vi "Create_LV_INI_Token.vi"   [LabVIEW 2021]
uses:
  <vilib>/Utility/config.llb/Write Key (String).vi
  <vilib>/Wiresmith Technology/G CLI/CLI Class/CLI.lvclass
  <vilib>/Utility/config.llb/NI_LVConfig.lvlib
types:
  T1 = enum32{"Invalid", "Standard", "Closed", "Hidden", "Minimized", "Maximized"}
  T2 = typedef "NI_LVConfig.lvlib/Config Data RefNum.ctl" = refnum<k1>
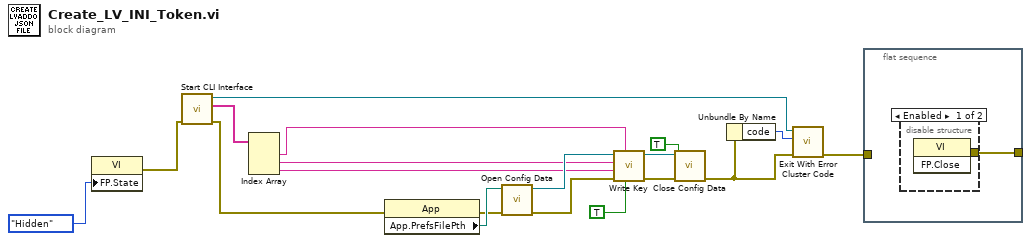
[diagram p0: block diagram]
diagram:
  n1 = property class="VI"("FP.State"=T1."Hidden" ("Front Panel Window:State")) -> (error out=w18:errorcluster)  [unwired: 2 in, 1 out]
  n2 = call <vilib>:"Start CLI Interface.vi"("error in (no error)"=w18) -> ("error out"=w8:errorcluster, "Custom Parameters"=w9:string[], "CLI out"=w16:refnum<class "CLI.lvclass">)  [unwired: 7 in, 1 out]
  n3 = Index Array(array=w9) -> (element #1=w5:string, element #2=w4:string, element #3=w3:string)  [unwired: 3 in]
  n4 = property class="App"(error in=w8) -> (error out=w12:errorcluster, "App.PrefsFilePth"=w15:path)  [unwired: 1 in, 1 out]
  n5 = call <vilib>:"Open Config Data.vi"("error in (no error)"=w12, "configuration file path"=w15) -> ("error out"=w13:errorcluster, "refnum"=w14:T2)  [unwired: 7 in, 1 out]
  n6 = call-poly <vilib>:"Write Key.vi"("write raw string? (F)"=TRUE, "section"=w5, "error in (no error)"=w13, "value"=w3, "key"=w4, "refnum"=w14) -> ("error out"=w11:errorcluster, "refnum out"=w10:T2)  [unwired: 3 in, 1 out]
  n7 = call <vilib>:"Close Config Data.vi"("error in (no error)"=w11, "write file if changed (T)"=TRUE, "refnum"=w10) -> ("error out"=w2:errorcluster)  [unwired: 7 in, 1 out]
  n8 = Unbundle By Name(w2) -> ("code"=w1:i32)
  n9 = call <vilib>:"Exit With Error Cluster Code.vi"("error in (no error)"=w2, "No Error Code (0)"=w1, "CLI in"=w16) -> ("error out"=w17:errorcluster)  [unwired: 8 in]
  n10 = flat-sequence {
    tunnel: [w20] -> _
    tunnel: w17 -> [_]
    frame #0 {
      n11 = disable-structure shown="Enabled" {
        disable-tunnel: [w21 _] -> w20
        frame Enabled {
          n12 = invoke class="VI" method="FP.Close"() -> (error out=w21:errorcluster)  [unwired: 3 in, 2 out]
        }
        frame Disabled {
        }
      }
    }
  }
